vi "Write Value (variant).vi"(8 "error in (no error)":errorcluster, 10 "Variant":variant, 11 "Bool D Element in":refnum<class "Bool D Element.lvclass">) -> (0 "error out":errorcluster, 3 "Bool D Element out":refnum<class "Bool D Element.lvclass">)   [LabVIEW 2018, in "D Datagrid Library.lvlib" / "Bool D Element.lvclass"]
uses:
  Bool D Element.lvclass
  Bool D Element.lvclass/Bool D Element.ctl
  Write Value.vi
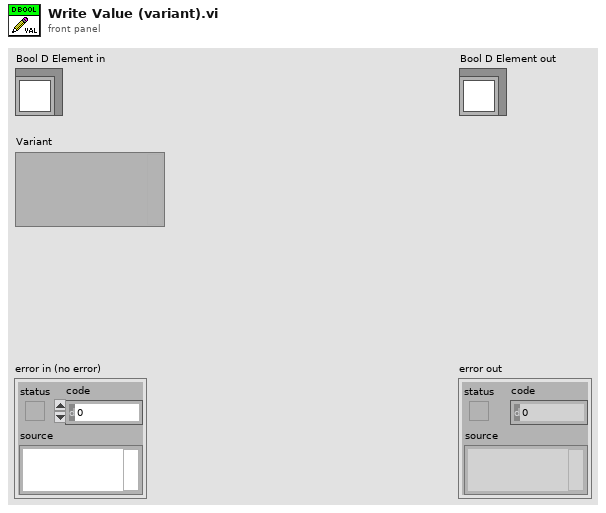
[diagram p1: front panel]
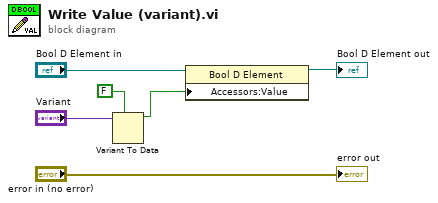
[diagram p0: block diagram]
diagram:
  n1 = Variant To Data(type=FALSE ("Value"), Variant="Variant") -> (data=w3:bool)  [unwired: 1 in, 1 out]
  n2 = property class="Bool D Element"(reference="Bool D Element in", "Accessors:Value"=w3) -> (reference out=→"Bool D Element out":refnum<class "Bool D Element.lvclass">)  [unwired: 1 in, 1 out]
  "error out" <- "error in (no error)"
